vi "open.vi"(8 "error in (no error)":errorcluster, 11 "Keysight 33500B in":refnum<class "Keysight 33511B.lvclass">) -> (0 "error out":errorcluster, 3 "Keysight 33500B out":refnum<class "Keysight 33511B.lvclass">)   [LabVIEW 2020, in "Keysight 33511B.lvclass"]
uses:
  Keysight 33511B.lvclass
  Keysight 33511B.lvclass/Keysight 33511B.ctl
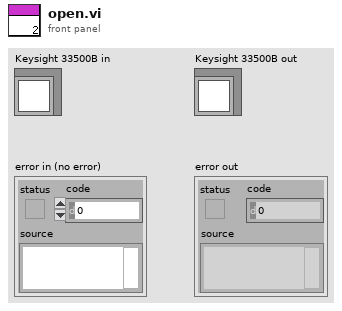
[diagram p1: front panel]
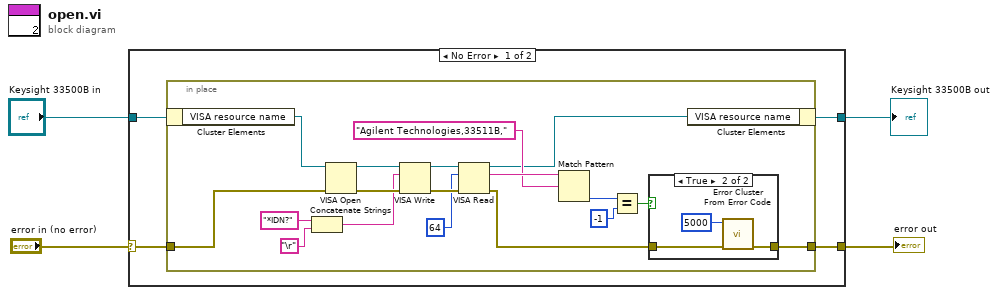
[diagram p0: block diagram]
diagram:
  n1 = case shown="No Error" "error in (no error)" {
    selector: "error in (no error)" -> [w7 w31]
    tunnel: "Keysight 33500B in" -> [w8 w32]
    tunnel: [w5 w32] -> w2
    tunnel: [w6 w31] -> w1
    frame No Error {
      n2 = in-place {
        in-place-border: w7 -> [w26]
        in-place-border: [w10] -> w6
        n3 = in-place-cluster #1(w8) -> ("VISA resource name"=w25:refnum<visa-resource-name>)
        n4 = Concatenate Strings("*IDN?", "\r") -> (w20:string)
        n5 = VISA Open(error in (no error)=w26, VISA resource name=w25) -> (VISA resource name=w24:refnum<visa-resource-name>, error out=w23:errorcluster)  [unwired: 3 in]
        n6 = VISA Write(VISA resource name=w24, write buffer=w20, error in (no error)=w23) -> (VISA resource name out=w18:refnum<visa-resource-name>, error out=w19:errorcluster)  [unwired: 1 out]
        n7 = VISA Read(VISA resource name=w18, byte count=u32 64, error in (no error)=w19) -> (VISA resource name out=w9:refnum<visa-resource-name>, read buffer=w13:string, error out=w11:errorcluster)  [unwired: 1 out]
        n8 = Match Pattern(string=w13, regular expression="Agilent Technologies,33511B,") -> (offset past match=w15:i32)  [unwired: 1 in, 3 out]
        n9 = Equal?(x=w15, y=-1) -> (x = y?=w16:bool)
        n10 = case shown="True" w16 {
          tunnel: w11 -> [w27 w29]
          tunnel: [w27 w28] -> w10
          frame False {
          }
          frame True {
            n11 = call <vilib>:"Error Cluster From Error Code.vi"("error in (no error)"=w29, "error code (0)"=5000) -> ("error out"=w28:errorcluster)  [unwired: 7 in]
          }
        }
        n12 = in-place-cluster #1("VISA resource name"=w9) -> (w5:refnum<class "Keysight 33511B.lvclass">)
      }
    }
    frame Error {
    }
  }
  "Keysight 33500B out" <- w2
  "error out" <- w1
